vi "Curtin_Undo.vi"(10 "New Files":T1[](array[typedef]), 11 "Array in":cluster{"files":T1[]}[](array[cluster])) -> (3 "Array out":cluster{"files":T1[]}[](array[cluster]))   [LabVIEW 2022 SP3]
uses:
  Curtin1_Label.ctl
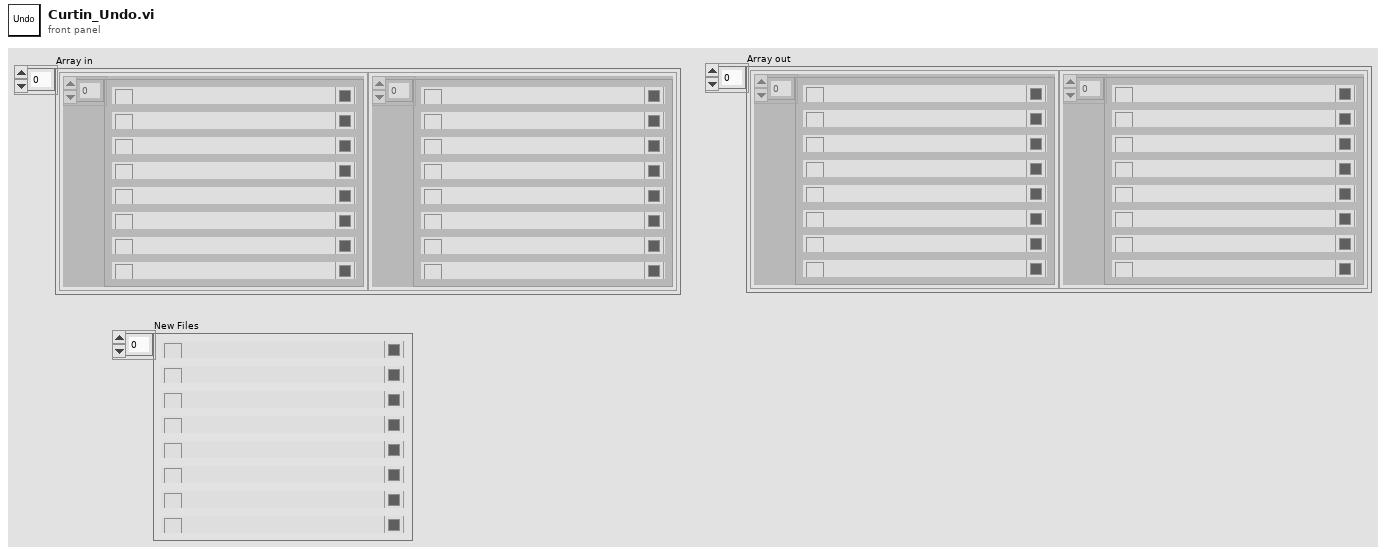
[diagram p1: front panel]
types:
  T1 = typedef "Curtin1_Label.ctl" = cluster{"Show?":bool, "Name":string, "Color":u32, "Path":path, "Show Notes":bool}
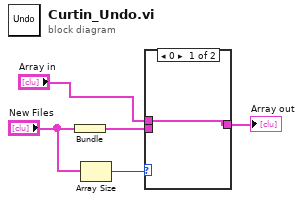
[diagram p0: block diagram]
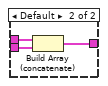
[diagram p2: hidden frame]
diagram:
  n1 = Bundle("New Files"="New Files") -> (w3:cluster{"New Files":T1[]})  [unwired: 1 in]
  n2 = Array Size(array="New Files") -> (size(s)=w1:i32)
  n3 = case shown="0" w1 {
    tunnel: [w6 w9] -> w5
    tunnel: "Array in" -> [w6 w8]
    tunnel: w3 -> [_ w7]
    frame 0 {
    }
    frame Default {
      n4 = Build Array (concatenate)(w8, w7) -> (w9:cluster{"New Files":T1[]}[])
    }
  }
  "Array out" <- w5
